vi "snap.vi"(8 "error in (no error)":errorcluster, 11 "camera in":refnum<class "camera.lvclass">) -> (0 "error out":errorcluster, 2 "Image Out":T1, 3 "camera out":refnum<class "camera.lvclass">)   [LabVIEW 2017, in "camera.lvclass"]
uses:
  camera.lvclass
  <vilib>/vision/Image Controls.llb/IMAQ Image.ctl
  <vilib>/vision/driver/IMAQdx.llb/IMAQdx Acquisition Mode.ctl
  <vilib>/vision/driver/IMAQdx.llb/IMAQdx Buffer Number Mode.ctl
  <vilib>/vision/driver/NI_Vision_Acquisition_Software.lvlib
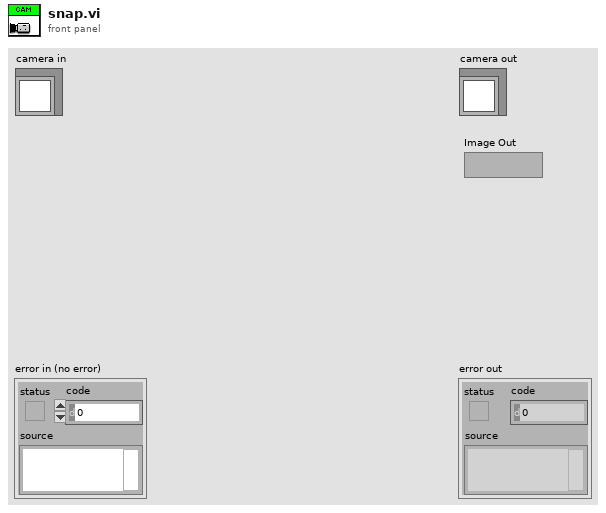
[diagram p1: front panel]
types:
  T1 = typedef "IMAQ Image.ctl" = refnum<image>
  T2 = typedef "NI_Vision_Acquisition_Software.lvlib/IMAQdx Buffer Number Mode.ctl" = enum32{"Next", "Last", "Buffer Number", "Every", "Last New"}
  T3 = typedef "NI_Vision_Acquisition_Software.lvlib/IMAQdx Acquisition Mode.ctl" = enum32{"One Shot", "Continuous"}
  T4 = typedef "IMAQdx.ctl" = refnum<k21>
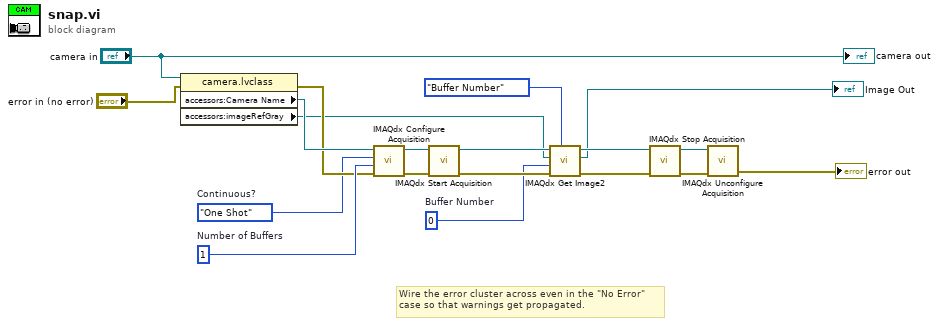
[diagram p0: block diagram]
diagram:
  w13 = u32 0  # Buffer Number
  w16 = u32 1  # Number of Buffers
  w4 = IMAQdx_Acquisition_Mode."One Shot"  # Continuous?
  # "Wire the error cluster across even in the \"No Error\"\ncase so that warnings get propagated."
  n1 = property class="camera.lvclass"(reference="camera in", error in="error in (no error)") -> (error out=w7:errorcluster, "accessors:Camera Name"=w8:refnum<k21>, "accessors:imageRefGray"=w2:T1)  [unwired: 1 out]
  n2 = call <vilib>:"IMAQdx Configure Acquisition.vi"("error in"=w7, "Number of Buffers"=w16, "Continuous?"=w4, "Session In"=w8) -> ("error out"=w18:errorcluster, "Session Out"=w12:T4)  [unwired: 6 out]
  n3 = call <vilib>:"IMAQdx Start Acquisition.vi"("error in"=w18, "Session In"=w12) -> ("error out"=w17:errorcluster, "Session Out"=w11:T4)  [unwired: 8 out]
  n4 = call <vilib>:"IMAQdx Get Image2.vi"("Buffer Number Mode (Next)"=IMAQdx_Buffer_Number_Mode."Buffer Number", "error in"=w17, "Buffer Number In"=w13, "Image In"=w2, "Session In"=w11) -> ("error out"=w14:errorcluster, "Image Out"=→"Image Out":T1, "Session Out"=w10:T4)  [unwired: 3 in, 1 out]
  n5 = call <vilib>:"IMAQdx Stop Acquisition.vi"("error in"=w14, "Session In"=w10) -> ("error out"=w15:errorcluster, "Session Out"=w9:T4)  [unwired: 8 out]
  n6 = call <vilib>:"IMAQdx Unconfigure Acquisition.vi"("error in"=w15, "Session In"=w9) -> ("error out"=→"error out":errorcluster)  [unwired: 9 out]
  "camera out" <- "camera in"
